vi "fpga_ARC FIFO control (32ch).vi"(7 "timestamp&count":T1 {"TAI timestamp" format="%.42g"}, 8 "Read FIFO":bool, 9 "write FIFO":bool, 10 "resample position":fxp<+,64,16> format="%.53g", 11 "frequency":fxp<+,32,8> format="%.27g") -> (0 "FIFO time out?":bool, 1 "timestamp&count":T1, 2 "resample position":fxp<+,64,16> format="%.53g", 3 "frequency":fxp<+,32,8> format="%.27g")   [LabVIEW 2014, in "NI_EP_Resample_FPGA.lvlib"]
uses:
  <vilib>/addons/Electrical Power/PQ/Resampling/NI_EP_Resample_FPGA.lvlib
  <vilib>/rvi/Emulation/niFpgaSctlEmulationGetInTimedLoop.vi
  <vilib>/rvi/DataTransferAndStorage/Container/Common/niFpgaContainerGetUniqueNameForEmu.vi
  <vilib>/rvi/DataTransferAndStorage/Container/Common/niFpgaContainerSetEmuInfo.vi
  <vilib>/rvi/eio/common/nirviEmuReportErrorAndStop.vi
  <vilib>/rvi/Emulation/niFpgaEmulationIsFPGAContextNoSignature.vi
  <vilib>/rvi/errors/niFpgaSetErrorForExecOnDevCompSimple.vi
  <vilib>/rvi/FIFO/Fifo_Resource/nirvififoEmulationSetSize.vi
  <vilib>/rvi/FIFO/Fifo_Resource/nirviFifoEmulationQueueMgr.vi
  <instcachedir>/0/nirviFifoEmulationQueueMgr_E5CAEC123FF24DC58D834DCA3CDAA9B5.lvgen/nirviFifoEmulationQueueMgr_E5CAEC123FF24DC58D834DCA3CDAA9B5_001.vi
  <vilib>/rvi/FIFO/Fifo_Resource/nirvififoEmulationCreateLock.vi
  <vilib>/rvi/Emulation/niFpgaProcessEmulError.vi
  <vilib>/rvi/FIFO/Fifo_Resource/nirvififoEmulationObtainLock.vi
  <vilib>/rvi/FIFO/Fifo_Resource/nirvififoEmulationReleaseLock.vi
  <vilib>/rvi/occurrence/nirviWaitOnOccurrenceBase.vi
  <vilib>/rvi/errors/nirviReportUnexpectedCaseInternalError.vi
  <vilib>/rvi/errors/nirviReportUnexpectedCaseInternalError (U32).vi
  <instcachedir>/0/nirviFifoEmulationQueueMgr_E5CAEC123FF24DC58D834DCA3CDAA9B5.lvgen/nirviFifoEmulationQueueMgr_E5CAEC123FF24DC58D834DCA3CDAA9B5_000.vi
  <instcachedir>/0/nirviFifoEmulationQueueMgr_E5CAEC123FF24DC58D834DCA3CDAA9B5.lvgen/nirviFifoEmulationQueueMgr_E5CAEC123FF24DC58D834DCA3CDAA9B5_009.vi
  <vilib>/rvi/FIFO/Fifo_Resource/nirvififoEmulationDetermineInputValidOut.vi
  <vilib>/rvi/LocalResourceManager/LocalResourceManager.xnode
  <vilib>/rvi/DataTransferAndStorage/Container/XNode/niFpgaContainer.xnode
  <vilib>/rvi/FIFO/Fifo_Resource/nirvififoEmulationRead.vi
  <vilib>/rvi/FIFO/Fifo_Resource/nirvififoEmulationWrite.vi
types:
  T1 = cluster{"TAI timestamp":fxp<+,64,32>, "AI Count":u16}
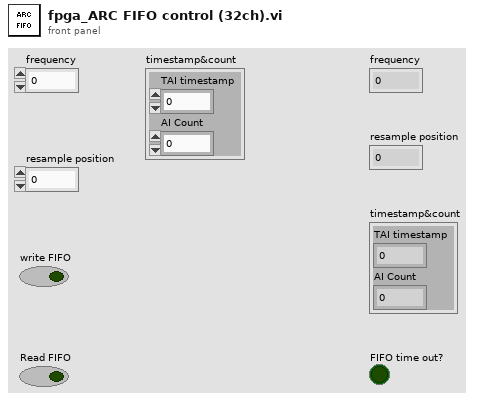
[diagram p1: front panel]
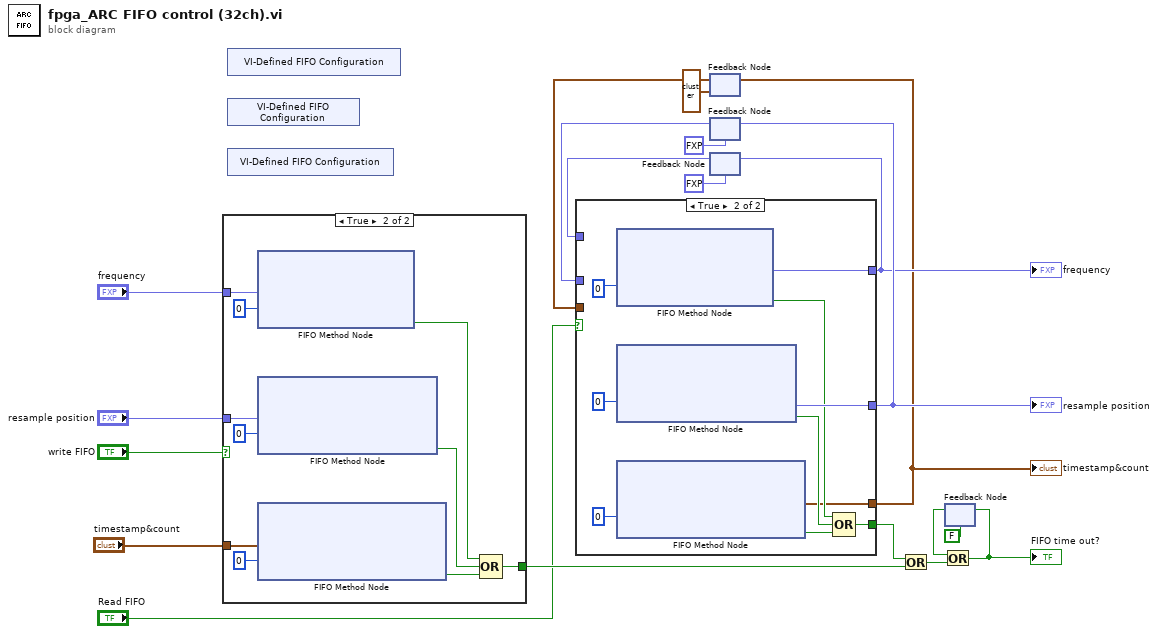
[diagram p0: block diagram]
diagram:
  n1 = case shown="True" "write FIFO" {
    tunnel: [_ w25] -> w20
    tunnel: "resample position" -> [_ w29]
    tunnel: "frequency" -> [_ w24]
    tunnel: "timestamp&count" -> [_ w21]
    frame False {
    }
    frame True {
      n2 = xnode ("FIFO Method Node")("Element"=w24, "Timeout"=0) -> ("Timed Out?"=w26:bool)  [unwired: 1 in, 1 out]
      n3 = xnode ("FIFO Method Node")("Element"=w29, "Timeout"=0) -> ("Timed Out?"=w27:bool)  [unwired: 1 in, 1 out]
      n4 = xnode ("FIFO Method Node")("Element"=w21, "Timeout"=0) -> ("Timed Out?"=w22:bool)  [unwired: 1 in, 1 out]
      n5 = Compound Arithmetic op=OR(w26, w27, w22) -> (w25:bool)
    }
  }
  n6 = xnode "VI-Defined FIFO Configuration"() -> ()  [unwired: 1 out]
  n7 = xnode "VI-Defined FIFO Configuration"() -> ()  [unwired: 1 out]
  n8 = xnode "VI-Defined FIFO Configuration"() -> ()  [unwired: 1 out]
  n9 = feedback #1(T1 {"TAI timestamp"=0.0, "AI Count"=0} ("Element")) -> (w2:T1)
  n10 = feedback #2(fxp<+,64,16> 0.0 ("Element")) -> (w18:fxp<+,64,16>)
  n11 = feedback #3(fxp<+,32,8> 0.0 ("Element")) -> (w16:fxp<+,32,8>)
  n12 = case shown="True" "Read FIFO" {
    tunnel: [w33 w42] -> w11
    tunnel: [_ w38] -> w19
    tunnel: w18 -> [w33 _]
    tunnel: [w32 w37] -> w9
    tunnel: w16 -> [w32 _]
    tunnel: [w31 w35] -> w3
    tunnel: w2 -> [w31 _]
    frame False {
    }
    frame True {
      n13 = xnode ("FIFO Method Node")("Timeout"=0) -> ("Element"=w37:fxp<+,32,8>, "Timed Out?"=w40:bool)  [unwired: 1 in, 1 out]
      n14 = xnode ("FIFO Method Node")("Timeout"=0) -> ("Element"=w42:fxp<+,64,16>, "Timed Out?"=w39:bool)  [unwired: 1 in, 1 out]
      n15 = xnode ("FIFO Method Node")("Timeout"=0) -> ("Element"=w35:T1, "Timed Out?"=w34:bool)  [unwired: 1 in, 1 out]
      n16 = Compound Arithmetic op=OR(w40, w39, w34) -> (w38:bool)
    }
  }
  "frequency" <- w9
  "resample position" <- w11
  "timestamp&count" <- w3
  n17 = feedback-in #1(w3) -> ()
  n18 = feedback-in #2(w11) -> ()
  n19 = feedback-in #3(w9) -> ()
  n20 = Or(x=w19, y=w20) -> (x .or. y?=w15:bool)
  n21 = feedback #4(FALSE) -> (w14:bool)
  n22 = Or(x=w14, y=w15) -> (x .or. y?=w12:bool)
  "FIFO time out?" <- w12
  n23 = feedback-in #4(w12) -> ()
